vi "i2c_osd_cmd_read.vi"(5 "COM":bool, 7 "VISA name":refnum<visa-resource-name>, 9 "data in":u8[](array[numeric]), 10 "byDataLen":u8, 11 "vdcmd_info_osd_t":T1) -> (2 "data out":u8[](array[numeric]), 3 "return":i32)   [LabVIEW 2016]
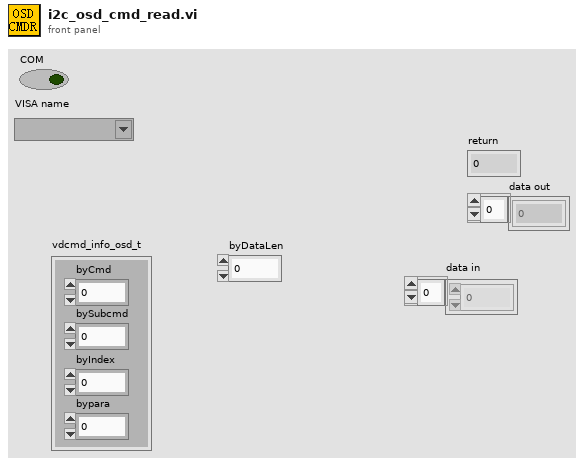
[diagram p1: front panel]
types:
  T1 = cluster{"byCmd":u8, "bySubcmd":u8, "byIndex":u8, "bypara":u8}
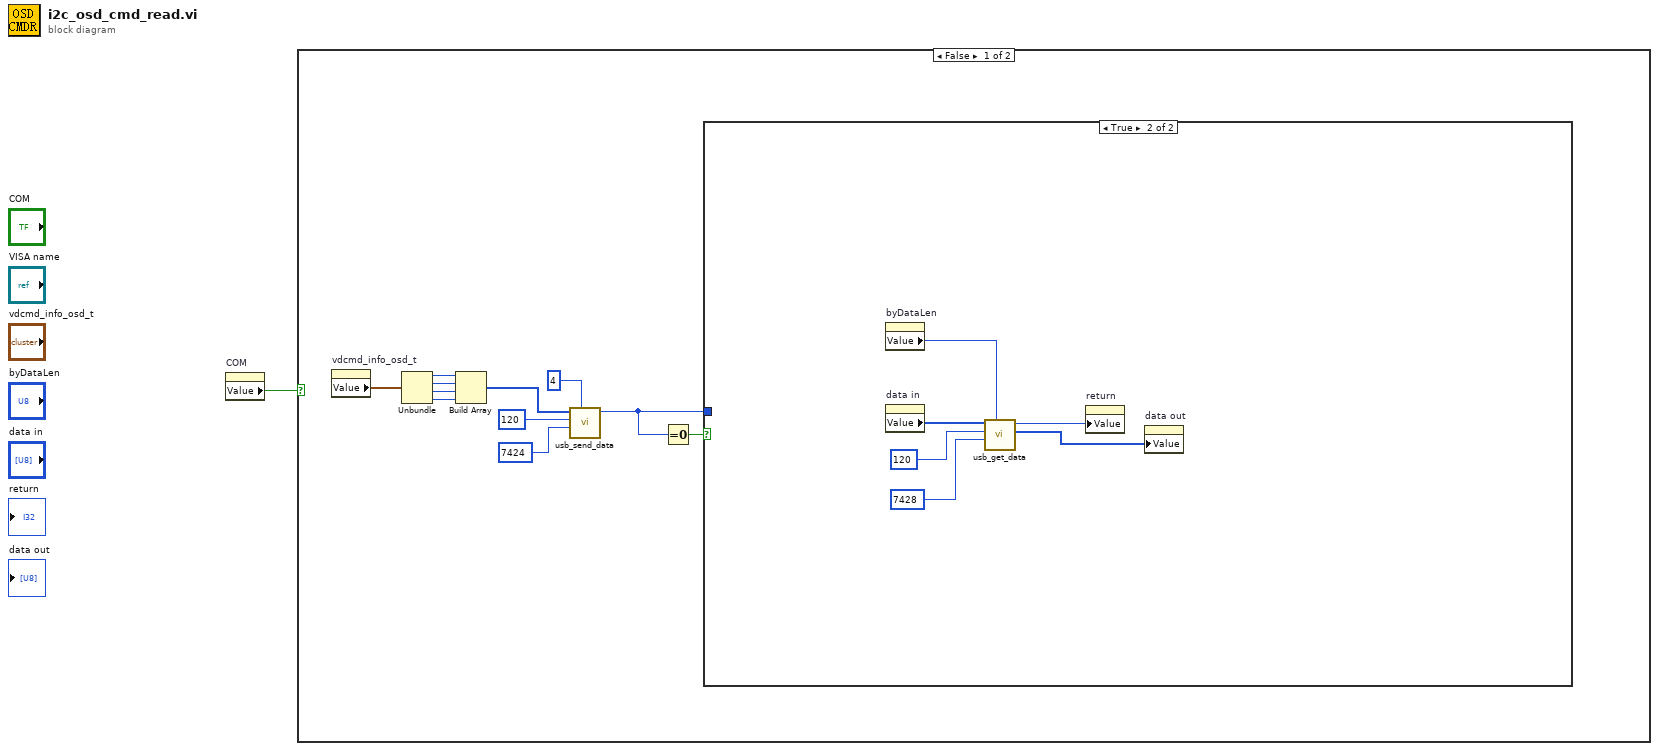
[diagram p0: block diagram]
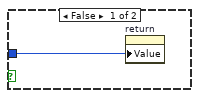
[diagram p2: hidden frame]
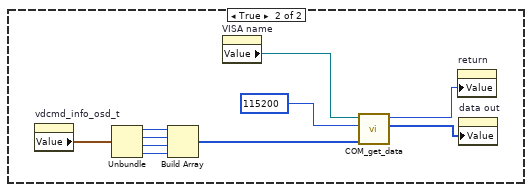
[diagram p3: hidden frame]
diagram:
  n1 = property on="COM" class="Bool (strict)"() -> ("Value"=w1:bool)  [unwired: 2 in, 2 out]
  n2 = case shown="False" w1 {
    frame False {
      n3 = property on="vdcmd_info_osd_t" class="Clust (strict)"() -> ("Value"=w11:T1)  [unwired: 2 in, 2 out]
      n4 = Unbundle(w11) -> ("byCmd"=w10:u8, "bySubcmd"=w9:u8, "byIndex"=w8:u8, "bypara"=w7:u8)
      n5 = Build Array(w10, w9, w8, w7) -> (w6:u8[])
      n6 = call "usb_send_data.vi"("byVdCmdHeaderLen"=u16 4, "I2C_VD_BUFFER_RW"=u16 7424, "I2C_SLAVE_ID"=u8 120, "data"=w6) -> ("return"=w2:i32)  [unwired: 6 in, 1 out]
      n7 = Equal To 0?(x=w2) -> (x = 0?=w3:bool)
      n8 = case shown="True" w3 {
        tunnel: w2 -> [w13 _]
        frame False {
          n9 = property on="return" class="DigNum (strict)"("Value"=w13) -> ()  [unwired: 2 in, 2 out]
        }
        frame True {
          n10 = property on="byDataLen" class="DigNum (strict)"() -> ("Value"=w18:u8)  [unwired: 2 in, 2 out]
          n11 = property on="data in" class="Arr (strict)"() -> ("Value"=w19:u8[])  [unwired: 2 in, 2 out]
          n12 = call "usb_get_data.vi"("byVdCmdHeaderLen"=w18, "I2C_VD_BUFFER_RW"=u16 7428, "I2C_SLAVE_ID"=u8 120, "data"=w19) -> ("data out"=w14:u8[], "return"=w15:i32)  [unwired: 5 in, 1 out]
          n13 = property on="return" class="DigNum (strict)"("Value"=w15) -> ()  [unwired: 2 in, 2 out]
          n14 = property on="data out" class="Arr (strict)"("Value"=w14) -> ()  [unwired: 2 in, 2 out]
        }
      }
    }
    frame True {
      n15 = property on="vdcmd_info_osd_t" class="Clust (strict)"() -> ("Value"=w26:T1)  [unwired: 2 in, 2 out]
      n16 = Unbundle(w26) -> ("byCmd"=w25:u8, "bySubcmd"=w24:u8, "byIndex"=w23:u8, "bypara"=w22:u8)
      n17 = Build Array(w25, w24, w23, w22) -> (w21:u8[])
      n18 = property on="VISA name" class="VISAName"() -> ("Value"=w27:refnum<visa-resource-name>)  [unwired: 2 in, 2 out]
      n19 = call "COM_get_data.vi"("data"=w21, "baud rate (9600)"=u32 115200, "VISA name"=w27) -> ("data out"=w29:u8[], "return"=w28:i32)  [unwired: 7 in]
      n20 = property on="return" class="DigNum (strict)"("Value"=w28) -> ()  [unwired: 2 in, 2 out]
      n21 = property on="data out" class="Arr (strict)"("Value"=w29) -> ()  [unwired: 2 in, 2 out]
    }
  }
